vi "Create.vi"(8 "error in (no error)":errorcluster, 11 "MB in":refnum<class "WebSocket Client CR.lvclass">) -> (0 "error out":errorcluster, 3 "MB out":refnum<class "WebSocket Client CR.lvclass">)   [LabVIEW 2021, in "WebSockets.lvlib" / "WebSocket Client CR.lvclass"]
uses:
  WebSocket Client CR.lvclass
  Master CR/Param/TCP Param/TCP Param.lvclass
  D:/my_projects/projects/Algorithms/Labview/21/Master CR/Param/Param.lvclass
  Data Model/WebSocket Data Model.lvclass
  D:/my_projects/projects/Algorithms/Labview/21/Modbus_v121c/Data Model/Device Data Model.lvclass
  ctl/Master CR state.ctl
  ctl/CR_Core_State.ctl
  WebSocket Client CR.lvclass/WebSocket Client CR.ctl
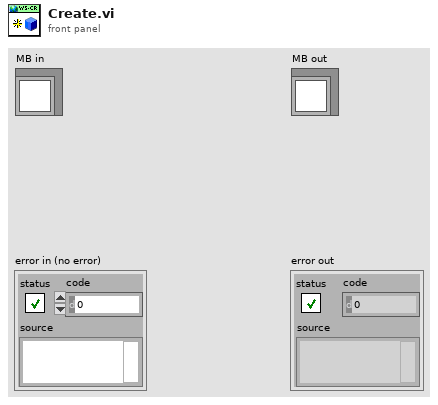
[diagram p1: front panel]
types:
  T1 = typedef "WebSockets.lvlib/WebSocket Client CR.lvclass/Master CR state.ctl" = cluster{"state":T2, "enable":bool, "write enable":bool, "connect":bool, "errors":i32, "Run":bool, "Write":bool, "Stop":bool}
  T2 = typedef "WebSockets.lvlib/WebSocket Client CR.lvclass/CR_Core_State.ctl" = enum8{"initialization", "redefine", "standby", "ping", "connect", "wait to reconnect", "wait to reset timeout", "configure", "requests", "close connection", "stop"}
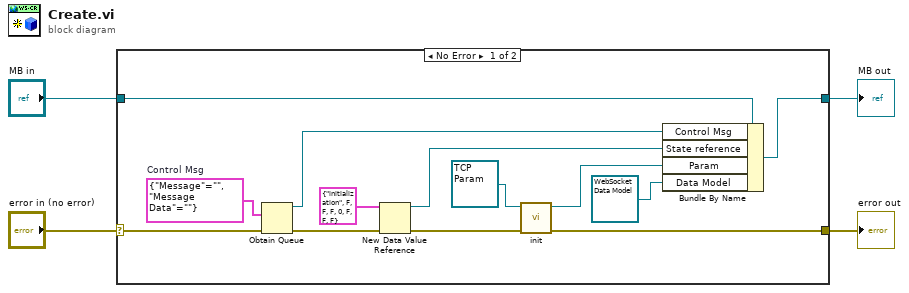
[diagram p0: block diagram]
diagram:
  n1 = case shown="No Error" "error in (no error)" {
    selector: "error in (no error)" -> [w10 w18]
    tunnel: "MB in" -> [w12 w19]
    tunnel: [w5 w18] -> w3
    tunnel: [w11 w19] -> w2
    frame No Error {
      w17 = cluster{"Message":string, "Message Data":string} {"Message"="", "Message Data"=""}  # Control Msg
      n2 = Obtain Queue(element data type=w17, error in (no error)=w10) -> (queue out=w14:refnum<queue>, error out=w13:errorcluster)  [unwired: 3 in, 1 out]
      n3 = New Data Value Reference(data value=T1 {"state"=enum."initialization", "enable"=FALSE, "write enable"=FALSE, "connect"=FALSE, "errors"=0, "Run"=FALSE, "Write"=FALSE, "Stop"=FALSE} ("State"), error in=w13) -> (data value reference=w15:refnum<data-value>, error out=w8:errorcluster)
      n4 = call-dynamic "init.vi"("error in"=w8, "Param in"=refnum<class "TCP Param.lvclass"> refnum ("Param.lvlib:TCP Param.lvclass")) -> ("error"=w5:errorcluster, "Param out"=w6:refnum<class "TCP Param.lvclass">)  [unwired: 8 in]
      n5 = Bundle By Name(cluster=w12, "Control Msg"=w14, "State reference"=w15, "Param"=w6, "Data Model"=refnum<class "WebSocket Data Model.lvclass"> refnum ("WebSockets.lvlib:Device Data Model")) -> (w11:refnum<class "WebSocket Client CR.lvclass">)
    }
    frame Error {
    }
  }
  "error out" <- w3
  "MB out" <- w2
